vi "Open in Explore.vi"(8 "error in (no error)":errorcluster, 11 "path":path) -> (0 "error out":errorcluster)   [LabVIEW 2019, in "Project Properties.lvlib"]
doc: "Opens the path in file explorer (Windows only).\n\nCreated by: Ryan Pacini"
uses:
  Project Properties.lvlib
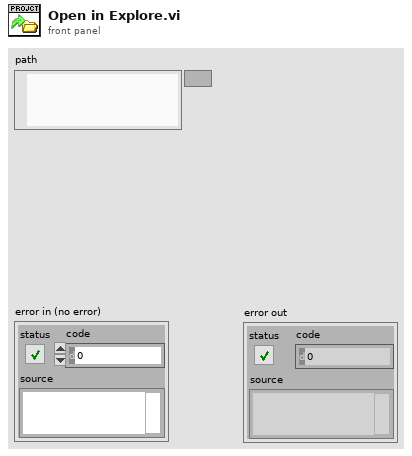
[diagram p1: front panel]
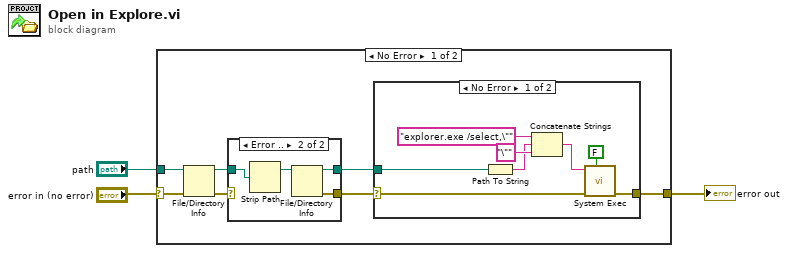
[diagram p0: block diagram]
diagram:
  n1 = case shown="No Error" "error in (no error)" {
    selector: "error in (no error)" -> [w6 w26]
    tunnel: "path" -> [w5 _]
    tunnel: [w4 w26] -> w1
    frame No Error {
      n2 = File/Directory Info(path=w5, error in=w6) -> (path out=w10:path, error out=w8:errorcluster)  [unwired: 5 out]
      n3 = case shown="Error .." w8 {
        selector: w8 -> [w11 _]
        tunnel: w10 -> [w12 w16]
        tunnel: [w11 w14] -> w9
        tunnel: [w12 w13] -> w7
        frame No Error {
        }
        frame Error {
          n4 = Strip Path(path=w16) -> (stripped path=w15:path)  [unwired: 1 out]
          n5 = File/Directory Info(path=w15) -> (path out=w13:path, error out=w14:errorcluster)  [unwired: 1 in, 5 out]
        }
      }
      n6 = case shown="No Error" w9 {
        selector: w9 -> [w17 w25]
        tunnel: [w19 w25] -> w4
        tunnel: w7 -> [w18 _]
        frame No Error {
          n7 = Path To String(path=w18) -> (string=w20:string)
          n8 = Concatenate Strings("explorer.exe /select,\"" ("string"), w20, "\"" ("string")) -> (w22:string)
          n9 = call <vilib>:"System Exec.vi"("wait until completion? (T)"=FALSE, "error in (no error)"=w17, "command line"=w22) -> ("error out"=w19:errorcluster)  [unwired: 5 in, 3 out]
        }
        frame Error {
        }
      }
    }
    frame Error {
    }
  }
  "error out" <- w1
